vi "Update In World.vi"(11 "Asteroid in":refnum<class "Planet.lvclass">) -> (3 "Asteroid out":refnum<class "Planet.lvclass">)   [LabVIEW 2015]
uses:
  Movable/Movable.lvclass
  <userlib>/_OpenG.lib/numeric/numeric.llb/Random Number Within Range - DBL__ogtk.vi
  Planet.lvclass
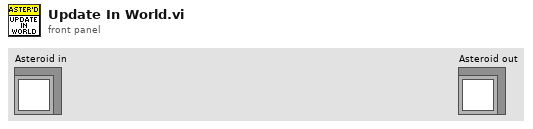
[diagram p1: front panel]
types:
  T1 = typedef "Constants.ctl" = cluster{"Colours":cluster{"OK":u32, "Warning":u32, "Error":u32, "Green On":u32, "Green Off":u32, "Red On":u32, "Red Off":u32}, "System":cluster{"Target Frames Second":dbl, "Field Size":T2, "Window Size":T2}, "Game":cluster{"Maximum Asteroids":i32}}
  T2 = typedef "Math.lvlib/Point (SGL).ctl" = cluster{"x":sgl, "y":sgl}
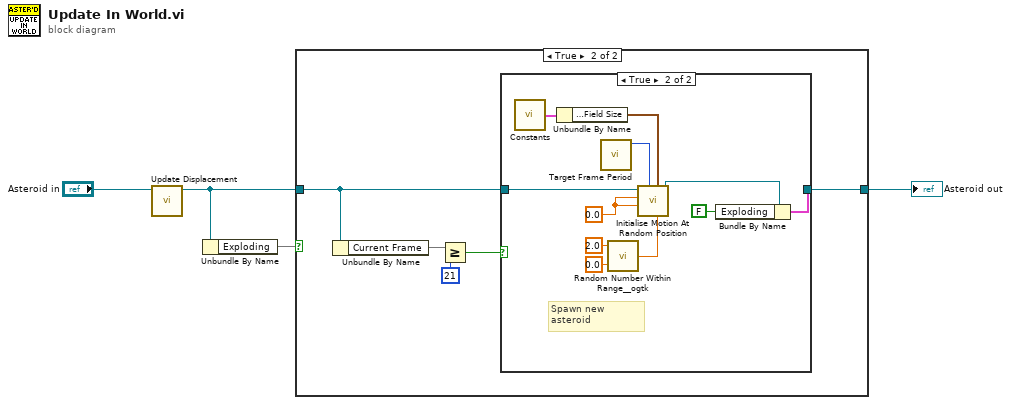
[diagram p0: block diagram]
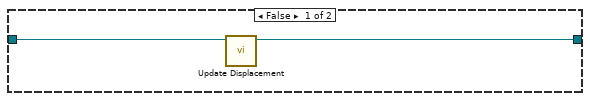
[diagram p2: hidden frame]
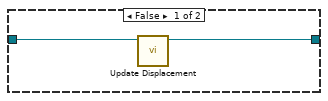
[diagram p3: hidden frame]
diagram:
  n1 = call "Update Displacement.vi"("Movable in"="Asteroid in") -> ("Movable out"=w2:refnum<class "Planet.lvclass">)  [unwired: 10 in]
  n2 = Unbundle By Name(w2) -> ("Exploding"=w3)
  n3 = case shown="True" w3 {
    tunnel: [w5 w8] -> w1
    tunnel: w2 -> [w6 w11]
    frame False {
      n4 = call "Update Displacement.vi"("Movable in"=w6) -> ("Movable out"=w5:refnum<class "Planet.lvclass">)  [unwired: 10 in]
    }
    frame True {
      n5 = Unbundle By Name(w11) -> ("Current Frame"=w7)
      n6 = Greater Or Equal?(x=w7, y=21) -> (x >= y?=w9:bool)
      n7 = case shown="True" w9 {
        tunnel: [w12 w15] -> w8
        tunnel: w11 -> [w13 w23]
        frame False {
          n8 = call "Update Displacement.vi"("Movable in"=w13) -> ("Movable out"=w12:refnum<class "Planet.lvclass">)  [unwired: 10 in]
        }
        frame True {
          w22 = sgl 0.0 ("Turn Rate [deg/s]")
          # "Spawn new asteroid"
          n9 = call "Constants.vi"() -> ("Constants"=w21:T1)
          n10 = Unbundle By Name(w21) -> ("System.Field Size"=w20:T2)
          n11 = call "Target Frame Period.vi"() -> ("Target Frame Period [ms]"=w24:u32)  [unwired: 11 in]
          n12 = call-poly <userlib>:"Random Number Within Range__ogtk.vi"("High"=sgl 2.0 ("Initial Heading [deg]"), "Low"=sgl 0.0 ("Initial Heading [deg]")) -> ("Random Number"=w17:dbl)  [unwired: 3 in]
          n13 = call "Initialise Motion At Random Position.vi"("Initial Velocity [m/s]"=w17, "Field Size"=w20, "Tick Period [ms]"=w24, "Thrust [m/s/s]"=w22, "Turn Rate [deg/s]"=w22, "Movable in"=w23) -> ("Movable out"=w16:refnum<class "Planet.lvclass">)  [unwired: 5 in]
          n14 = Bundle By Name(cluster=w16, "Exploding"=FALSE) -> (w15:cluster{})
        }
      }
    }
  }
  "Asteroid out" <- w1
